vi "detect motion 1.vi"(10 "thresh 1":refnum<vi>, 11 "external stop":refnum<vi>) -> ()   [LabVIEW 2013]
uses:
  <vilib>/vision/NI_Vision_Development_Module.lvlib
panel:
  out "integral":u32[][](array[numeric])
  out "motionpix1":refnum<queue>
  out "Waveform Chart 2":i32(graph)=500
  out "Particle Measurements (Pixels)":dbl[][](array[numeric])=[[1238.5, 0.5, 8.0], [1396.0, 0.5, 6.0], [1625.0, 0.5, 6.0], [1729.0, 0.5, 6.0], [2493.0, 0.5, 6.0], [1720.0, 15.0, 9.0], [655.0, 58.0, 9.0], [967.0, 58.0, 9.0], [1103.0, 61.0, 9.0], [1898.0, 76.0, 9.0], [1755.0, 88.0, 9.0], [1493.0, 89.0, 9.0], [1605.0, 99.0, 9.0], [1760.0, 100.0, 9.0], [651.0, 105.0, 9.0], [1684.0, 113.0, 9.0], [2265.0, 119.0, 9.0], [2126.0, 120.0, 9.0], [1463.0, 122.0, 9.0], [914.0, 175.0, 9.0], [337.5, 177.0, 12.0], [1450.0, 177.0, 9.0], [1274.0, 180.0, 9.0], [1741.0, 185.0, 9.0], [1371.0, 193.0, 9.0], [1723.0, 197.0, 9.0], [2478.0, 197.0, 9.0], [1557.0, 198.0, 9.0], [1478.0, 205.0, 9.0], [1712.0, 213.0, 9.0], [2130.5, 216.0, 12.0], [1757.0, 218.0, 9.0], [1509.0, 224.0, 9.0], [1311.0, 226.0, 9.0], [1155.0, 239.5, 12.0], [1614.0, 256.0, 9.0], [1886.0, 267.0, 9.0], [749.0, 274.0, 9.0], [1444.0, 281.0, 9.0], [712.0, 285.0, 9.0], [1672.0, 285.0, 9.0], [1184.0, 303.0, 9.0], [2038.0, 315.0, 9.0], [2056.0, 319.0, 9.0], [2312.0, 321.0, 9.0], [1082.0, 330.0, 9.0], [2391.0, 332.0, 9.0], [1053.0, 335.0, 9.0], [1622.0, 338.0, 9.0], [2555.0, 338.0, 9.0], [2367.0, 344.0, 9.0], [1400.0, 350.0, 9.0], [1497.0, 354.0, 9.0], [1293.0, 369.0, 9.0], [2538.0, 372.0, 9.0], [921.0, 375.0, 9.0], [2551.0, 376.0, 9.0], [879.0, 377.0, 9.0], [1374.0, 385.0, 9.0], [1105.0, 404.0, 9.0], [1638.0, 410.0, 9.0], [1006.0, 411.0, 9.0], [1373.0, 432.5, 12.0], [1713.0, 439.0, 9.0], [1022.0, 440.0, 9.0], [787.0, 455.0, 9.0], [899.0, 457.0, 9.0], [1631.0, 460.0, 9.0], [2005.0, 463.0, 9.0], [1672.0, 464.0, 9.0], [1724.0, 465.0, 9.0], [1157.5, 473.0, 12.0], [1274.0, 474.0, 9.0], [2451.0, 476.0, 9.0], [1756.0, 480.0, 9.0], [1711.0, 481.0, 9.0], [1346.0, 485.0, 9.0], [1986.0, 485.0, 9.0], [1373.0, 488.0, 9.0], [1752.0, 499.0, 9.0], [2493.0, 500.0, 9.0], [2048.0, 501.0, 9.0], [1032.0, 505.0, 9.0], [1745.0, 510.0, 9.0], [1031.0, 511.0, 9.0], [2175.0, 511.0, 9.0], [2193.0, 512.0, 9.0], [822.0, 519.0, 9.0], [2192.0, 527.0, 9.0], [1689.0, 531.0, 9.0], [1379.0, 532.0, 9.0], [1511.5, 540.0, 12.0], [387.0, 541.0, 9.0], [1221.5, 543.0, 12.0], [2180.0, 548.0, 9.0], [1514.0, 553.0, 9.0], [1285.0, 555.0, 9.0], [2003.0, 555.0, 9.0], [1041.0, 561.5, 12.0], [506.0, 565.0, 9.0], [1933.0, 567.0, 9.0], [1029.0, 571.0, 9.0], [1201.0, 571.0, 9.0], [2235.0, 572.0, 9.0], [1188.0, 576.5, 12.0], [1584.0, 578.0, 9.0], [1148.0, 587.0, 9.0], [891.0, 590.0, 9.0], [674.5, 591.0, 12.0], [2214.0, 594.0, 9.0], [1906.0, 596.0, 9.0], [1675.0, 601.0, 9.0], [1104.0, 602.5, 12.0], [1794.5, 602.0, 12.0], [1218.0, 605.0, 9.0], [1835.0, 611.0, 9.0], [1623.0, 612.0, 9.0], [1335.0, 616.0, 9.0], [733.0, 617.5, 12.0], [1031.0, 622.0, 9.0], [1779.0, 627.0, 9.0], [1155.0, 640.0, 9.0], [1147.5, 642.5, 14.0], [1904.0, 642.0, 9.0], [791.0, 647.0, 9.0], [1400.0, 647.0, 9.0], [1804.0, 650.0, 9.0], [1894.0, 650.0, 9.0], [1547.0, 655.0, 9.0], [1372.0, 658.0, 9.0], [460.0, 659.0, 9.0], [1645.0, 660.5, 12.0], [1267.0, 661.5, 12.0], [2131.0, 661.0, 9.0], [1475.0, 664.0, 9.0], [472.0, 671.0, 9.0], [1735.0, 680.7142857142857, 21.0], [811.0, 684.0, 9.0], [1489.0, 688.0, 9.0], [1631.0, 694.0, 9.0], [2494.5, 698.0, 12.0], [1065.0, 701.0, 9.0], [698.0, 704.0, 9.0], [1900.0, 704.0, 9.0], [2273.0, 706.0, 9.0], [1815.0, 708.0, 9.0], [1600.0, 710.5, 12.0], [1111.0, 712.5, 12.0], [1346.0, 715.0, 9.0], [1496.0, 717.0, 9.0], [1236.0, 719.0, 9.0], [2146.0, 720.0, 9.0], [1548.0, 727.0, 9.0], [1539.0, 729.0, 9.0], [1189.0, 735.5, 12.0], [1571.0, 736.0, 9.0], [1242.5, 737.0, 12.0], [2010.0, 743.0, 9.0], [1543.0, 746.0, 9.0], [1695.0, 746.0, 9.0], [956.0, 747.0, 9.0], [1675.0, 749.0, 9.0], [1485.0, 754.0, 9.0], [1953.0, 754.0, 9.0], [1084.0, 755.0, 9.0], [1984.0, 757.0, 9.0], [1692.0, 759.0, 9.0], [1994.0, 761.0, 9.0], [1367.0, 769.0, 9.0], [1554.0, 769.0, 9.0], [957.0, 770.0, 9.0], [1646.0, 777.5, 12.0], [1933.0, 778.0, 9.0], [1532.0, 779.0, 9.0], [1849.0, 779.0, 9.0], [1310.0, 782.0, 9.0], [1733.0, 786.0, 9.0], [1477.0, 789.0, 9.0], [890.0, 792.0, 9.0], [2526.0, 792.0, 9.0], [1317.0, 795.0, 9.0], [2334.0, 796.0, 9.0], [1410.0, 812.0, 9.0], [1058.0, 813.0, 9.0], [1305.0, 820.0, 9.0], [2127.0, 820.0, 9.0], [539.0, 825.0, 9.0], [2329.0, 825.0, 9.0], [1025.0, 826.0, 9.0], [1079.0, 828.0, 9.0], [1829.0, 839.0, 9.0], [2265.0, 841.0, 9.0], [1950.0, 843.0, 9.0], [2440.0, 849.0, 9.0], [539.0, 850.0, 9.0], [1719.0, 854.0, 9.0], [2357.0, 854.0, 9.0], [1083.0, 858.0, 9.0], [1114.0, 860.0, 9.0], [1915.0, 868.0, 9.0], [2095.0, 869.5, 12.0], [2182.0, 870.0, 9.0], [1713.0, 874.5, 12.0], [1011.0, 877.0, 9.0], [1695.0, 877.0, 9.0], [1883.0, 878.0, 9.0], [2207.0, 879.5, 12.0], [2287.0, 880.0, 9.0], [413.0, 882.0, 9.0], [1209.0, 886.0, 9.0], [1648.0, 891.0, 9.0], [1917.0, 894.0, 9.0], [2447.0, 894.0, 9.0], [904.0, 899.0, 9.0], [2203.0, 899.0, 9.0], [1996.0, 900.0, 9.0], [2306.0, 900.0, 9.0], [1433.0, 906.0, 9.0], [2346.0, 906.0, 9.0], [2086.0, 911.0, 9.0], [2005.0, 912.5, 12.0], [1055.0, 921.0, 9.0], [2206.0, 923.0, 9.0], [1642.0, 927.0, 9.0], [871.0, 929.5, 12.0], [1650.5, 929.0, 12.0], [2219.0, 932.0, 9.0], [1534.5, 933.0, 12.0], [1487.0, 939.0, 9.0], [803.0, 943.0, 9.0], [2321.0, 945.0, 9.0], [1693.0, 951.0, 9.0], [1621.0, 953.0, 9.0], [1725.0, 963.0, 9.0], [1759.0, 964.0, 9.0], [2051.0, 966.0, 9.0], [160.0, 972.0, 9.0], [385.0, 973.0, 9.0], [2514.0, 974.0, 9.0], [1228.0, 976.0, 9.0], [2145.0, 982.0, 9.0], [993.0, 986.0, 9.0], [1134.0, 990.0, 9.0], [1650.0, 990.0, 9.0], [2411.0, 991.0, 9.0], [666.0, 992.0, 9.0], [945.0, 993.0, 9.0], [988.0, 993.0, 9.0], [1369.0, 993.0, 9.0], [1519.0, 994.0, 9.0], [995.0, 995.5, 12.0], [1331.0, 1002.0, 9.0], [1353.0, 1002.0, 9.0], [2175.0, 1005.0, 9.0], [1000.0, 1006.5, 12.0], [2302.0, 1008.0, 9.0], [956.0, 1015.0, 9.0], [2245.0, 1015.5, 12.0], [2396.0, 1018.0, 9.0], [1378.0, 1020.0, 9.0], [858.0, 1023.0, 9.0], [1142.0, 1023.0, 9.0], [1662.0, 1023.0, 9.0], [1171.0, 1025.0, 9.0], [2191.0, 1026.0, 9.0], [1295.0, 1027.0, 9.0], [1000.0, 1028.0, 9.0], [1593.0, 1029.0, 9.0], [1079.0, 1031.0, 9.0], [369.0, 1032.0, 9.0], [1836.0, 1033.0, 9.0], [1648.0, 1044.0, 9.0], [1726.0, 1044.0, 9.0], [2495.0, 1045.0, 9.0], [1582.0, 1048.0, 9.0], [2238.0, 1052.0, 9.0], [0.5, 1054.0, 6.0], [949.6, 1054.4, 15.0], [1226.0, 1056.0, 9.0], [2164.0, 1056.0, 9.0], [2005.5, 1059.0, 12.0], [408.0, 1066.0, 9.0], [1065.0, 1077.5, 12.0], [1805.0, 1081.0, 9.0], [1871.0, 1087.0, 9.0], [1138.0, 1091.0, 9.0], [1572.0, 1091.0, 9.0], [2288.0, 1092.0, 9.0], [1060.0, 1096.0, 9.0], [2377.5, 1103.0, 12.0], [2566.0, 1103.0, 9.0], [1078.0, 1107.0, 9.0], [1017.5, 1110.0, 12.0], [1180.0, 1113.0, 9.0], [240.0, 1124.0, 9.0], [1463.0, 1132.0, 9.0], [2232.0, 1132.0, 9.0], [1443.0, 1140.0, 9.0], [2259.0, 1142.0, 9.0], [1238.0, 1143.5, 12.0], [1874.0, 1145.0, 9.0], [437.0, 1148.0, 9.0], [1315.0, 1153.0, 9.0], [2548.0, 1155.0, 15.0], [1118.0, 1157.0, 9.0], [1437.0, 1163.0, 9.0], [1433.0, 1169.0, 9.0], [2049.0, 1169.0, 9.0], [2228.5, 1169.0, 12.0], [954.0, 1170.5, 12.0], [1734.5, 1170.0, 12.0], [1969.0, 1171.0, 9.0], [1908.0, 1172.0, 9.0], [2374.0, 1175.0, 9.0], [2502.0, 1175.0, 9.0], [2052.0, 1178.0, 9.0], [2229.0, 1181.0, 9.0], [2166.0, 1188.0, 9.0], [2280.0, 1189.0, 9.0], [1054.0, 1190.5, 12.0], [2443.0, 1191.0, 9.0], [1253.0, 1192.0, 9.0], [1326.0, 1192.0, 9.0], [2092.0, 1192.0, 9.0], [1257.0, 1193.0, 9.0], [1998.0, 1197.0, 9.0], [2208.5, 1199.0, 12.0], [1233.0, 1201.0, 9.0], [1831.0, 1204.0, 9.0], [1731.0, 1209.0, 9.0], [2246.0, 1213.0, 9.0], [770.5, 1215.0, 12.0], [1424.0, 1216.0, 9.0], [2516.0, 1219.0, 9.0], [1973.0, 1224.0, 9.0], [2146.9411764705883, 1226.5882352941176, 17.0], [778.0, 1227.0, 9.0], [896.0, 1228.0, 9.0], [1585.0, 1228.0, 9.0], [2332.0, 1228.0, 9.0], [2019.0, 1233.0, 9.0], [2257.0, 1233.0, 9.0], [2022.0, 1240.0, 9.0], [1524.0, 1242.0, 9.0], [2399.0, 1247.0, 9.0], [1378.4, 1251.4, 15.0], [1971.0, 1252.0, 9.0], [1100.5, 1255.0, 12.0], [1942.0, 1255.0, 9.0], [1916.0, 1258.0, 9.0], [912.0, 1262.0, 9.0], [1928.0, 1262.0, 9.0], [1469.0, 1265.0, 9.0], [1240.0, 1270.0, 9.0], [1790.5, 1277.0, 12.0], [2043.0, 1278.0, 9.0], [2306.0, 1278.0, 9.0], [1209.0, 1281.0, 9.0], [1369.0, 1283.0, 9.0], [1051.0, 1284.0, 9.0], [1092.0, 1317.0, 9.0], [1596.0, 1320.0, 9.0], [847.0, 1321.5, 12.0], [1315.0, 1322.0, 15.0], [1462.0, 1321.5, 12.0], [1900.0, 1341.0, 9.0], [2377.0, 1341.0, 9.0], [2460.0, 1349.0, 9.0], [2506.0, 1349.0, 9.0], [711.0, 1351.0, 9.0], [1717.0, 1354.0, 9.0], [1064.0, 1356.0, 9.0], [1000.0, 1359.0, 9.0], [1959.0, 1362.0, 15.0], [1820.0, 1362.0, 9.0], [1856.0, 1366.0, 9.0], [1925.0, 1367.0, 9.0], [1106.0, 1371.0, 9.0], [2237.0, 1377.0, 9.0], [1612.0, 1382.0, 9.0], [1954.0, 1383.0, 9.0], [1859.5, 1384.0, 12.0], [2234.0, 1387.0, 9.0], [2244.0, 1388.0, 9.0], [1166.0, 1391.0, 9.0], [1059.5, 1394.0, 12.0], [2044.0, 1394.0, 9.0], [1985.0, 1396.0, 9.0], [754.0, 1397.0, 9.0], [1479.0, 1398.0, 9.0], [1813.0, 1398.0, 9.0], [973.0, 1401.0, 9.0], [2455.0, 1406.0, 9.0], [1945.6, 1408.6, 15.0], [2041.0, 1412.0, 9.0], [2324.0, 1416.0, 9.0], [2284.0, 1417.0, 9.0], [2428.0, 1419.0, 9.0], [1115.0, 1420.0, 9.0], [2059.0, 1420.0, 9.0], [1609.0, 1423.0, 9.0], [1906.0, 1432.0, 9.0], [1125.0, 1434.0, 9.0], [1252.0, 1440.0, 9.0], [1711.0, 1444.0, 9.0], [2244.0, 1444.0, 9.0], [1238.0, 1456.0, 9.0], [1788.0, 1458.0, 9.0], [1052.0, 1461.0, 9.0], [2547.5, 1463.0, 12.0], [1812.0, 1467.5, 12.0], [2061.0, 1468.0, 9.0], [1511.0, 1470.0, 9.0], [1495.0, 1478.0, 9.0], [1103.0, 1483.0, 9.0], [1820.0, 1486.0, 9.0], [2398.0, 1486.0, 9.0], [2249.0, 1489.0, 9.0], [1719.0, 1490.0, 9.0], [1743.0, 1494.0, 9.0], [1986.0, 1495.0, 9.0], [769.0, 1502.0, 9.0], [2422.0, 1502.0, 9.0], [2395.0, 1509.0, 9.0], [593.0, 1510.0, 9.0], [2111.0, 1516.0, 9.0], [2547.0, 1519.0, 9.0], [1573.0, 1524.0, 9.0], [1340.0, 1525.0, 9.0], [1173.0, 1528.0, 9.0], [2338.0, 1531.0, 9.0], [456.5, 1541.0, 12.0], [1971.5, 1542.0, 12.0], [933.0, 1548.0, 9.0], [1228.0, 1555.0, 9.0], [1934.0, 1559.0, 9.0], [1961.0, 1559.0, 9.0], [2487.0, 1560.0, 9.0], [1070.0, 1566.0, 9.0], [1023.0, 1567.0, 9.0], [2208.0, 1567.0, 9.0], [2376.5, 1567.0, 12.0], [2090.0, 1569.0, 9.0], [1946.0, 1570.0, 9.0], [2234.0, 1571.0, 9.0], [1840.0, 1572.0, 9.0], [819.0, 1574.0, 9.0], [1180.0, 1578.5, 12.0], [1733.0, 1580.0, 9.0], [2073.0, 1585.0, 9.0], [2250.0, 1590.0, 9.0], [2345.0, 1590.0, 9.0], [1008.0, 1595.0, 9.0], [1367.0, 1596.0, 9.0], [2215.5, 1602.0, 12.0], [2129.0, 1612.0, 9.0], [1288.0, 1614.0, 9.0], [1715.0, 1615.0, 9.0], [1573.0, 1625.0, 9.0], [2057.0, 1640.0, 9.0], [2117.0, 1642.0, 9.0], [670.0, 1643.0, 9.0], [2461.5, 1647.0, 12.0], [1971.0, 1665.0, 9.0], [1682.0, 1666.0, 9.0], [975.0, 1679.0, 9.0], [2444.0, 1682.0, 9.0], [1513.0, 1687.0, 9.0], [1080.0, 1690.0, 9.0], [2153.0, 1699.0, 9.0], [1546.0, 1701.0, 9.0], [2005.0, 1709.0, 9.0], [1229.0, 1712.0, 9.0], [2460.0, 1725.0, 9.0], [380.0, 1732.0, 9.0], [2251.0, 1736.0, 9.0], [2477.0, 1737.0, 9.0], [1313.0, 1741.0, 9.0], [1645.0, 1750.0, 9.0], [2139.0, 1752.0, 9.0], [1233.0, 1772.0, 9.0], [1156.0, 1793.0, 9.0], [1749.0, 1806.0, 9.0], [1831.0, 1811.0, 9.0], [2451.0, 1821.0, 9.0], [1636.0, 1847.0, 9.0], [1819.0, 1852.5, 12.0], [2288.0, 1856.0, 9.0], [1507.0, 1864.0, 9.0], [1485.0, 1876.0, 9.0], [700.0, 1881.0, 9.0], [1788.0, 1898.0, 9.0], [1292.0, 1915.0, 9.0], [1360.0, 1934.0, 9.0], [743.0, 1942.5, 6.0], [783.0, 1942.5, 6.0], [1038.0, 1942.5, 6.0], [1843.0, 1942.5, 6.0], [1959.0, 1942.5, 6.0], [2084.0, 1942.5, 6.0]] format="%.2f"
  in  "Pixel Measurements":T1[](array[typedef])=[0, 1, 35] items=["Center of Mass X", "Center of Mass Y", "First Pixel X", "First Pixel Y", "Bounding Rect Left", "Bounding Rect Top", "Bounding Rect Right", "Bounding Rect Bottom", "Max Feret Diameter Start X", "Max Feret Diameter Start Y", "Max Feret Diameter End X", "Max Feret Diameter End Y", "Max Horiz. Segment Length Left", "Max Horiz. Segment Length Right", "Max Horiz. Segment Length Row", "-", "Bounding Rect Width", "Bounding Rect Height", "Bounding Rect Diagonal", "Perimeter", "Convex Hull Perimeter", "Holes' Perimeter", "Max Feret Diameter", "Equivalent Ellipse Major Axis", "Equivalent Ellipse Minor Axis", "Equivalent Ellipse Minor Axis (Feret)", "Equivalent Rect Long Side", "Equivalent Rect Short Side", "Equivalent Rect Diagonal", "Equivalent Rect Short Side (Feret)", "Average Horiz. Segment Length", "Average Vert. Segment Length", "Hydraulic Radius", "Waddel Disk Diameter", "-", "Area", "Holes' Area", "Particle & Holes' Area", "Convex Hull Area", "Image Area", "-", "Number of Holes", "Number of Horiz. Segments", "Number of Vert. Segments", "-", "Orientation", "Max Feret Diameter Orientation", "-", "% Area/Image Area", "% Area/(Particle & Holes' Area)", "Ratio of Equivalent Ellipse Axes", "Ratio of Equivalent Rect Sides", "-", "Elongation Factor", "Compactness Factor", "Heywood Circularity Factor", "Type Factor", "-", "Sum X", "Sum Y", "Sum XX", "Sum XY", "Sum YY", "Sum XXX", "Sum XXY", "Sum XYY", "Sum YYY", "-", "Moment of Inertia XX", "Moment of Inertia XY", "Moment of Inertia YY", "Moment of Inertia XXX", "Moment of Inertia XXY", "Moment of Inertia XYY", "Moment of Inertia YYY", "Norm. Moment of Inertia XX", "Norm. Moment of Inertia XY", "Norm. Moment of Inertia YY", "Norm. Moment of Inertia XXX", "Norm. Moment of Inertia XXY", "Norm. Moment of Inertia XYY", "Norm. Moment of Inertia YYY", "Hu Moment 1", "Hu Moment 2", "Hu Moment 3", "Hu Moment 4", "Hu Moment 5", "Hu Moment 6", "Hu Moment 7"]
  out "error out":errorcluster
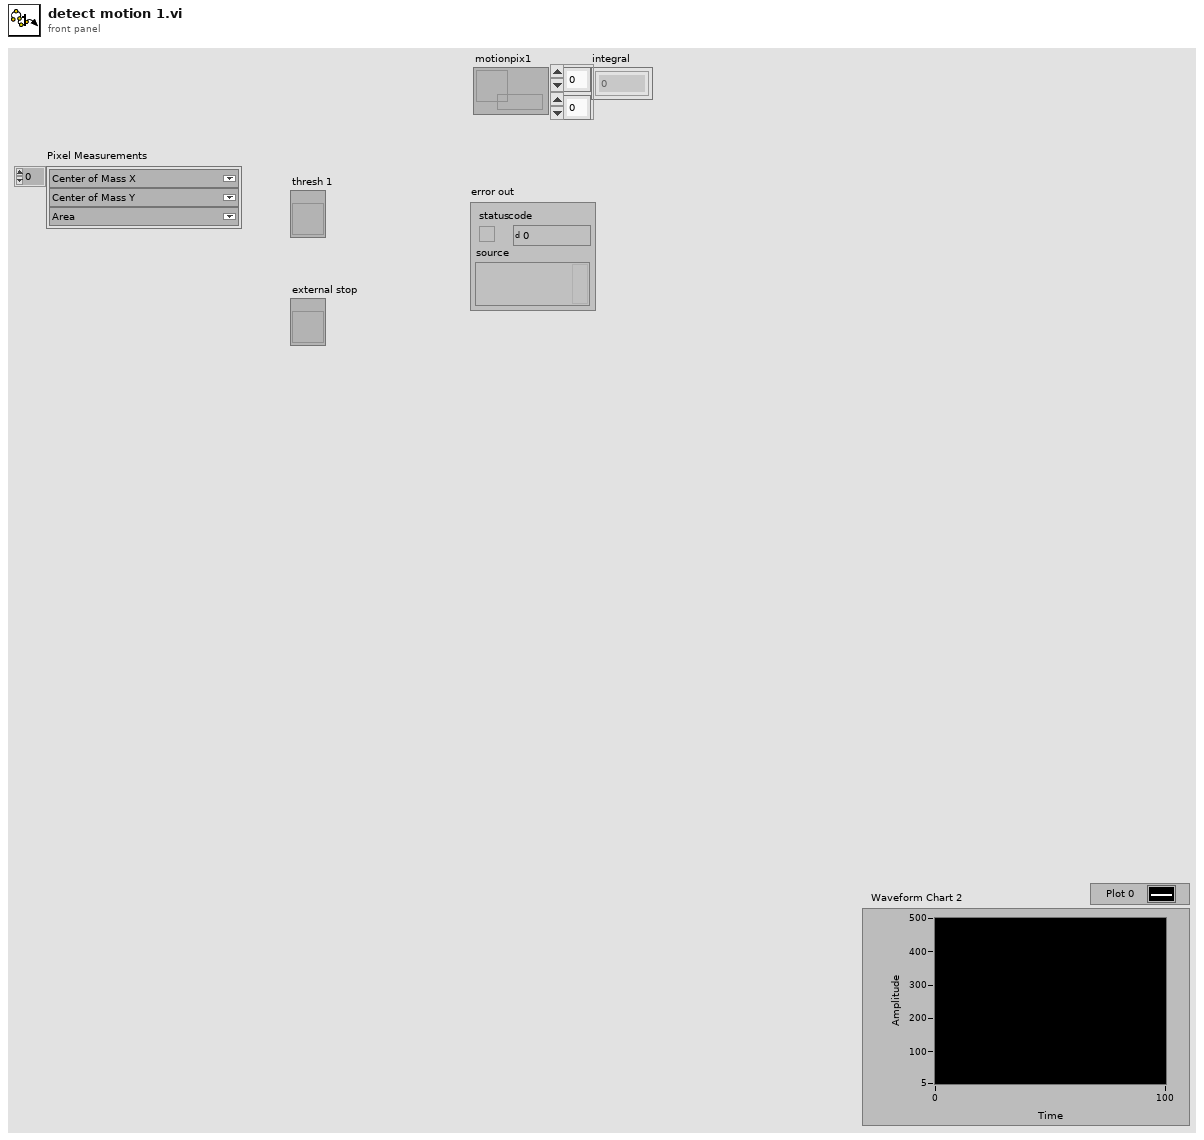
[diagram p1: front panel]
types:
  T1 = typedef "Particle Parameters" = i32
  T2 = typedef "Image Type" = u32
  T3 = typedef "IMAQ Image.ctl" = refnum<image>
  T4 = enum32{"AutoM", "Close", "Dilate", "Erode", "Gradient", "Gradient out", "Gradient in", "Hit miss", "Open", "PClose", "POpen", "Thick", "Thin"}
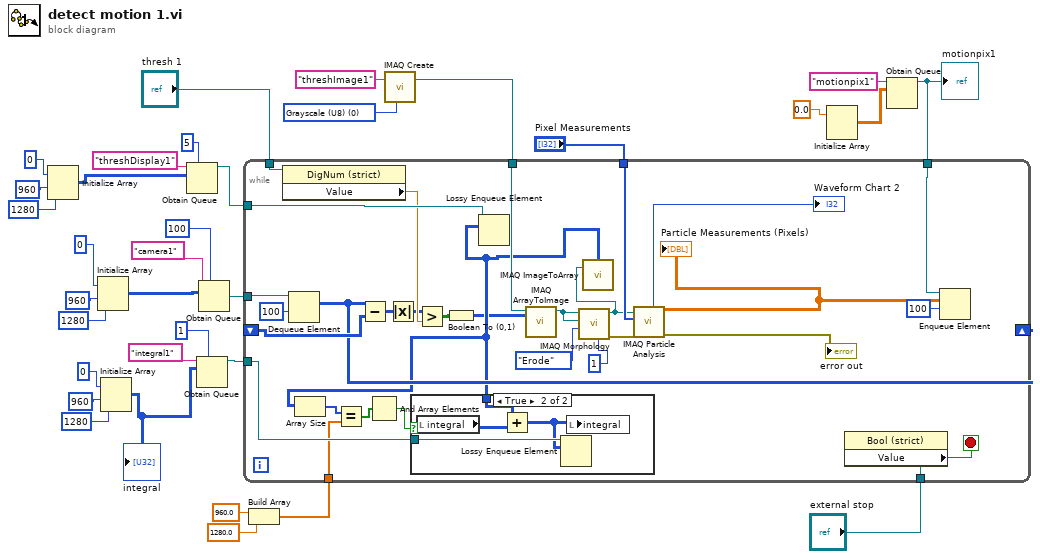
[diagram p0: block diagram]
diagram:
  w27 = T2 0 items=["Grayscale (U8)", "Grayscale (I16)", "Grayscale (SGL)", "Complex (CSG)", "RGB (U32)", "HSL (U32)", "RGB (U64)", "Grayscale (U16)"] ("Image Type")
  n1 = Initialize Array(u8 0 ("element"), 960 ("dimension size"), 1280 ("dimension size")) -> (w11:u8[][])
  n2 = Initialize Array(i16 0 ("element"), 960 ("dimension size"), 1280 ("dimension size")) -> (w18:i16[][])
  n3 = Initialize Array(u32 0 ("element"), 960 ("dimension size"), 1280 ("dimension size")) -> (w4:u32[][])
  "integral" <- w4
  n4 = Obtain Queue(max queue size (-1, unlimited)=5, name (unnamed)="threshDisplay1", element data type=w11) -> (queue out=w17:refnum<queue>)  [unwired: 2 in, 2 out]
  n5 = Obtain Queue(max queue size (-1, unlimited)=1, name (unnamed)="integral1", element data type=w4) -> (queue out=w5:refnum<queue>)  [unwired: 2 in, 2 out]
  n6 = Obtain Queue(max queue size (-1, unlimited)=100, name (unnamed)="camera1", element data type=w18) -> (queue out=w34:refnum<queue>)  [unwired: 2 in, 2 out]
  n7 = Build Array(960.0 ("element"), 1280.0 ("element")) -> (w1:dbl[])
  n8 = call "IMAQ Create"("Image Name"="threshImage1", "Image Type"=w27) -> ("New Image"=w28:T3)  [unwired: 3 in, 1 out]
  n9 = Initialize Array(0.0 ("element")) -> (w23:dbl[][])  [unwired: 2 in]
  n10 = Obtain Queue(name (unnamed)="motionpix1", element data type=w23) -> (queue out=w21:refnum<queue>)  [unwired: 3 in, 2 out]
  "motionpix1" <- w21
  n11 = while {
    tunnel: w34 -> [w65]
    tunnel: w28 -> [w60]
    shift-right: [w51] -> _
    shift-left: _ -> [w63]
    tunnel: "Pixel Measurements" -> [w62]
    tunnel: "external stop" -> [w59]
    tunnel: w21 -> [w57]
    tunnel: w17 -> [w54]
    tunnel: "thresh 1" -> [w53]
    tunnel: w5 -> [w50]
    tunnel: w1 -> [w47]
    stop <- w58 stop-if-true
    n12 = property class="DigNum (strict)"(reference=w53) -> ("Value"=w52:dbl)  [unwired: 1 in, 2 out]
    n13 = Dequeue Element(queue=w65, timeout in ms (-1)=100) -> (element=w51:i16[][])  [unwired: 1 in, 3 out]
    n14 = Subtract(x=w51, y=w63) -> (x-y=w37:i16[][])
    n15 = Absolute Value(x=w37) -> (abs(x)=w36:i16[][])
    n16 = Greater?(x=w36, y=w52) -> (0:w35:bool[][])
    n17 = Boolean To (0,1)(Boolean=w35) -> (0, 1=w43:i16[][])
    n18 = call "IMAQ ArrayToImage"("Image Pixels (U8)"=w43, "Image"=w60) -> ("Image Out"=w40:T3)  [unwired: 8 in, 1 out]
    n19 = call "IMAQ Morphology"("Number of iterations (1)"=1, "Operation"=T4."Erode", "Image Dst"=w40, "Image Src"=w40) -> ("error out"=w39:errorcluster, "Image Dst Out"=w38:T3)  [unwired: 6 in]
    n20 = call "IMAQ ImageToArray"("Image"=w38) -> ("Image Pixels (U8)"=w49:u8[][])  [unwired: 3 in, 4 out]
    n21 = Array Size(array=w49) -> (size(s)=w48:i32[])
    n22 = Equal?(x=w48, y=w47) -> (x = y?=w46:bool[])
    n23 = And Array Elements(Boolean array=w46) -> (logical AND=w45:bool)
    n24 = case shown="True" w45 {
      tunnel: w50 -> [_ w69]
      tunnel: w49 -> [_ w66]
      frame False {
      }
      frame True {
        n25 = local read "integral"() -> (w68:u32[][])
        n26 = Add(x=w66, y=w68) -> (x+y=w67:u32[][])
        n27 = Lossy Enqueue Element(queue=w69, element=w67) -> ()  [unwired: 1 in, 4 out]
        n28 = local write "integral"(w67) -> ()
      }
    }
    n29 = Lossy Enqueue Element(queue=w54, element=w49) -> ()  [unwired: 1 in, 4 out]
    n30 = call "IMAQ Particle Analysis"("error in (no error)"=w39, "Pixel Measurements"=w62, "Image"=w38) -> ("error out"=→"error out":errorcluster, "Particle Measurements (Pixels)"=w56:dbl[][], "Number of Particles"=→"Waveform Chart 2":i32)  [unwired: 3 in, 3 out]
    "Particle Measurements (Pixels)" <- w56
    n31 = property class="Bool (strict)"(reference=w59) -> ("Value"=w58:bool)  [unwired: 1 in, 2 out]
    n32 = Enqueue Element(queue=w57, element=w56, timeout in ms (-1)=100) -> ()  [unwired: 1 in, 3 out]
  }
